vi "Write_Header_Erd_Name_&_Number.vi"(0 "Refnum_In_Csv":refnum<file>, 5 "Write_Header?":bool, 7 "ERD Name Array In":string[](array[string]), 9 "ERD Number Array In":string[](array[string])) -> (4 "Refnum_Out_Csv":refnum<file>)   [LabVIEW 2023]
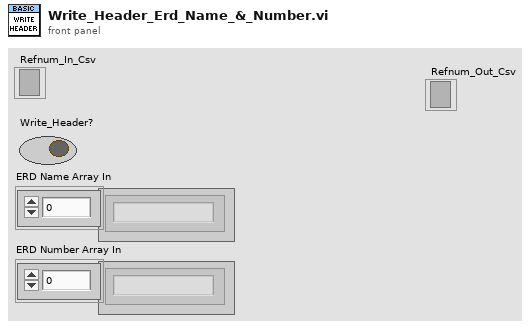
[diagram p1: front panel]
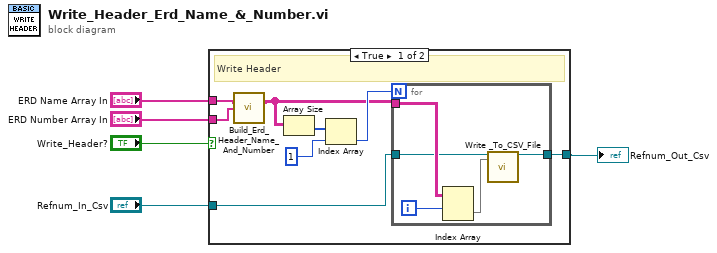
[diagram p0: block diagram]
diagram:
  n1 = case shown="True" "Write_Header?" {
    tunnel: [w13 w19] -> w1
    tunnel: "ERD Name Array In" -> [w8 _]
    tunnel: "ERD Number Array In" -> [w7 _]
    tunnel: "Refnum_In_Csv" -> [w6 w19]
    frame True {
      # "Write Header"
      n2 = call "Build_Erd_Header_Name_And_Number.vi"("ERD Name Array In"=w8, "ERD Number Array In"=w7) -> ("Header_To_Write"=w9:string[][])  [unwired: 13 in]
      n3 = Array Size(array=w9) -> (size(s)=w12:i32[])
      n4 = Index Array(array=w12, index=1) -> (element=w10:i32)
      n5 = for {
        N: w10 -> [_]
        tunnel: [w18] -> w13
        tunnel: w9 -> [w17]
        tunnel: w6 -> [w14]
        i -> [w16]
        n6 = Index Array(array=w17, index (row)=w16) -> (element=w15:string[])  [unwired: 1 in]
        n7 = call "Write _To_CSV_File.vi"("Refnum In"=w14, "ERD Name"=w15) -> ("Refnum Out"=w18:refnum<file>)  [unwired: 15 in, 2 out]
      }
    }
    frame False {
    }
  }
  "Refnum_Out_Csv" <- w1
